vi "SCPI.Send.vi"(8 "error in (no error)":errorcluster, 10 "SCPI command":string, 11 "Instrument.SCPI in":refnum<class "Instrument.SCPI.lvclass">) -> (0 "error out":errorcluster, 3 "Instrument.SCPI out":refnum<class "Instrument.SCPI.lvclass">)   [LabVIEW 2019, in "Instrument.SCPI.lvclass"]
uses:
  Instrument.SCPI.lvclass
  C:/Users/patrick/Documents/GitHub/Instrument-Framework/lvsrc/Framework/Instrument/Instrument.lvclass
  Typedefs/SCPI.Commands--Enum.ctl
  Instrument/Instrument.lvclass
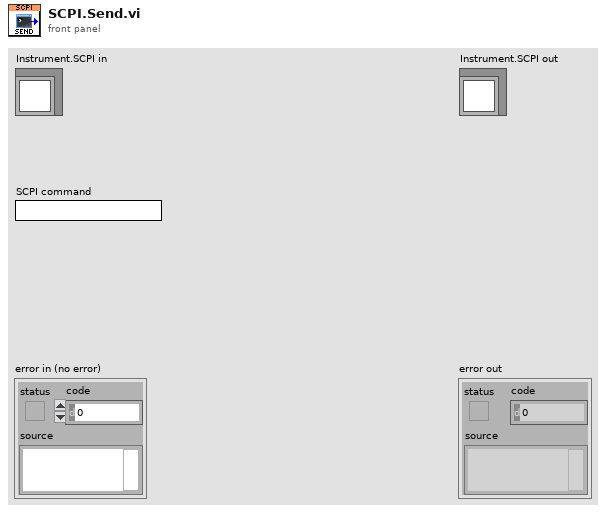
[diagram p1: front panel]
types:
  T1 = typedef "Instrument.SCPI.lvclass/SCPI.Commands--Enum.ctl" = enum16{"sendSCPI", "receiveSCPI"}
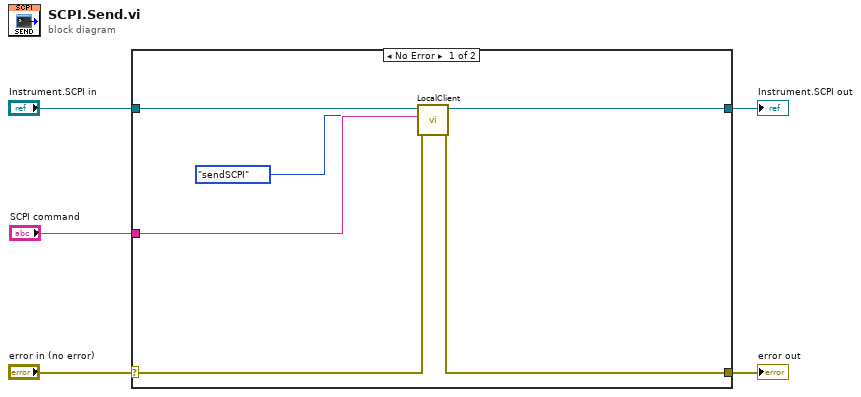
[diagram p0: block diagram]
diagram:
  n1 = case shown="No Error" "error in (no error)" {
    selector: "error in (no error)" -> [w6 w13]
    tunnel: [w9 w13] -> w5
    tunnel: [w10 w12] -> w3
    tunnel: "Instrument.SCPI in" -> [w11 w12]
    tunnel: "SCPI command" -> [w8 _]
    frame No Error {
      n2 = call "LocalClient.vi"("timeout (ms) [500]"=SCPI.Commands--Enum."sendSCPI" ("Commands"), "error in (no error)"=w6, "Command in"=w8, "Instrument in"=w11) -> ("error out"=w9:errorcluster, "Instrument out"=w10:refnum<class "Instrument.SCPI.lvclass">)  [unwired: 4 in, 2 out]
    }
    frame Error {
    }
  }
  "error out" <- w5
  "Instrument.SCPI out" <- w3
